vi "DownsampleStage3_x410_10MHzPID.vi"(6 "Count to skip":u32=22, 8 "valid in":bool, 9 "reset":bool, 11 "Data in":fxp<+/-,32,14>[](array[numeric])=[0.0, 0.0, 0.0, 0.0, 0.0, 0.0]) -> (0 "valid out":bool, 3 "data out":fxp<+/-,32,14>[](array[numeric]))   [LabVIEW 2025]
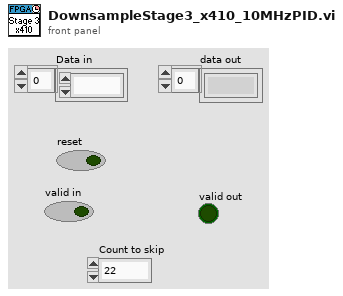
[diagram p1: front panel]
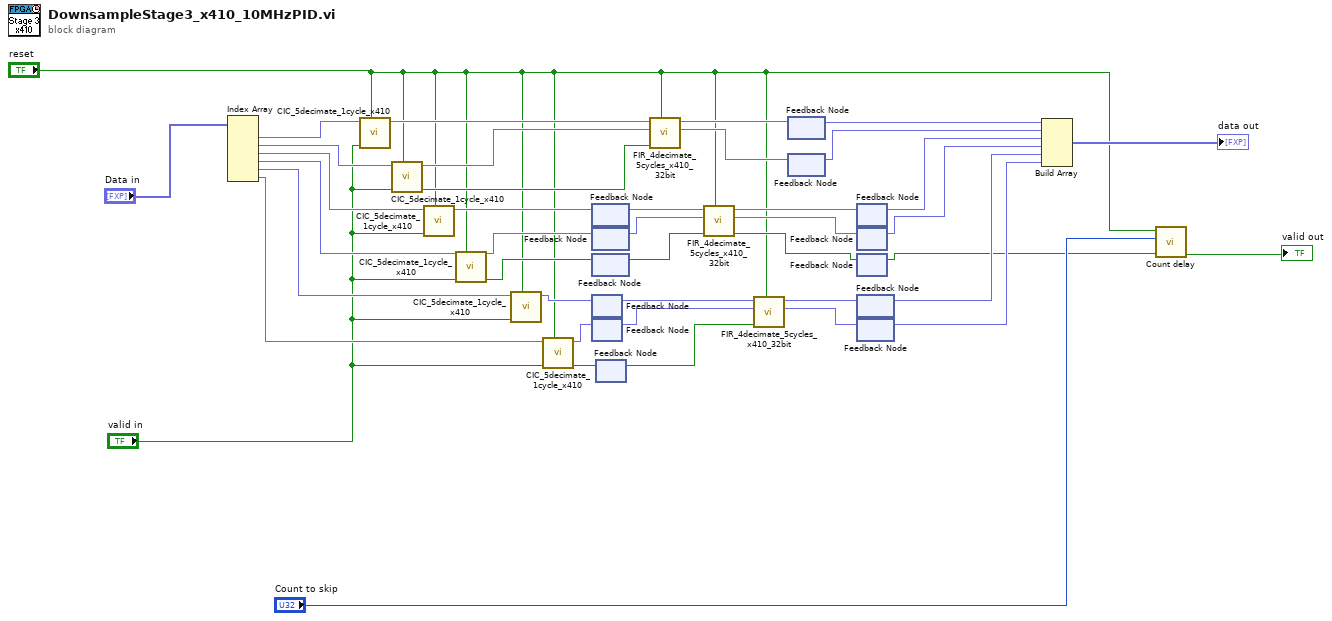
[diagram p0: block diagram]
diagram:
  n1 = Index Array(array="Data in") -> (element #1=w40:fxp<+/-,32,14>, element #2=w38:fxp<+/-,32,14>, element #3=w37:fxp<+/-,32,14>, element #4=w36:fxp<+/-,32,14>, element #5=w17:fxp<+/-,32,14>, element #6=w16:fxp<+/-,32,14>)  [unwired: 6 in]
  n2 = call "CIC_5decimate_1cycle_x410.vi"("reset"="reset", "valid in"="valid in", "Data in"=w40) -> ("Data out"=w29:fxp<+/-,32,14>)  [unwired: 7 in, 1 out]
  n3 = call "CIC_5decimate_1cycle_x410.vi"("reset"="reset", "valid in"="valid in", "Data in"=w38) -> ("valid out"=w27:bool, "Data out"=w28:fxp<+/-,32,14>)  [unwired: 7 in]
  n4 = call "CIC_5decimate_1cycle_x410.vi"("reset"="reset", "valid in"="valid in", "Data in"=w37) -> ("Data out"=w35:fxp<+/-,32,14>)  [unwired: 7 in, 1 out]
  n5 = call "CIC_5decimate_1cycle_x410.vi"("reset"="reset", "valid in"="valid in", "Data in"=w36) -> ("valid out"=w33:bool, "Data out"=w34:fxp<+/-,32,14>)  [unwired: 7 in]
  n6 = call "CIC_5decimate_1cycle_x410.vi"("reset"="reset", "valid in"="valid in", "Data in"=w17) -> ("Data out"=w11:fxp<+/-,32,14>)  [unwired: 7 in, 1 out]
  n7 = call "CIC_5decimate_1cycle_x410.vi"("reset"="reset", "valid in"="valid in", "Data in"=w16) -> ("valid out"=w7:bool, "Data out"=w10:fxp<+/-,32,14>)  [unwired: 7 in]
  n8 = feedback #1() -> (w32:fxp<+/-,32,14>)  [unwired: 1 in]
  n9 = feedback-in #1(w35) -> ()
  n10 = feedback #2() -> (w31:fxp<+/-,32,14>)  [unwired: 1 in]
  n11 = feedback-in #2(w34) -> ()
  n12 = feedback #3() -> (w30:bool)  [unwired: 1 in]
  n13 = feedback-in #3(w33) -> ()
  n14 = feedback #4() -> (w12:fxp<+/-,32,14>)  [unwired: 1 in]
  n15 = feedback-in #4(w11) -> ()
  n16 = feedback #5() -> (w13:fxp<+/-,32,14>)  [unwired: 1 in]
  n17 = feedback-in #5(w10) -> ()
  n18 = feedback #6() -> (w6:bool)  [unwired: 1 in]
  n19 = feedback-in #6(w7) -> ()
  n20 = call "FIR_4decimate_5cycles_x410_32bit.vi"("reset"="reset", "valid in"=w27, "Q in"=w28, "I in"=w29) -> ("Q out"=w25:fxp<+/-,32,14>, "I out"=w26:fxp<+/-,32,14>)  [unwired: 4 in, 2 out]
  n21 = call "FIR_4decimate_5cycles_x410_32bit.vi"("reset"="reset", "valid in"=w30, "Q in"=w31, "I in"=w32) -> ("valid out"=w20:bool, "Q out"=w21:fxp<+/-,32,14>, "I out"=w22:fxp<+/-,32,14>)  [unwired: 4 in, 1 out]
  n22 = call "FIR_4decimate_5cycles_x410_32bit.vi"("reset"="reset", "valid in"=w6, "Q in"=w13, "I in"=w12) -> ("Q out"=w15:fxp<+/-,32,14>, "I out"=w14:fxp<+/-,32,14>)  [unwired: 4 in, 2 out]
  n23 = feedback #7() -> (w24:fxp<+/-,32,14>)  [unwired: 1 in]
  n24 = feedback-in #7(w26) -> ()
  n25 = feedback #8() -> (w23:fxp<+/-,32,14>)  [unwired: 1 in]
  n26 = feedback-in #8(w25) -> ()
  n27 = feedback #9() -> (w18:fxp<+/-,32,14>)  [unwired: 1 in]
  n28 = feedback-in #9(w22) -> ()
  n29 = feedback #10() -> (w19:fxp<+/-,32,14>)  [unwired: 1 in]
  n30 = feedback-in #10(w21) -> ()
  n31 = feedback #11() -> (w3:bool)  [unwired: 1 in]
  n32 = feedback-in #11(w20) -> ()
  n33 = feedback #12() -> (w9:fxp<+/-,32,14>)  [unwired: 1 in]
  n34 = feedback-in #12(w14) -> ()
  n35 = feedback #13() -> (w8:fxp<+/-,32,14>)  [unwired: 1 in]
  n36 = feedback-in #13(w15) -> ()
  n37 = Build Array(w24, w23, w18, w19, w9, w8) -> (→"data out":fxp<+/-,32,14>[])
  n38 = call "Count delay.vi"("input valid"=w3, "Count to skip"="Count to skip", "Reset"="reset") -> ("output valid"=→"valid out":bool)  [unwired: 7 in, 1 out]
